vi "McPherson Set Scanning.vi"(0 "VISA Resource Name":refnum<visa-resource-name>, 1 "Stop@End?":bool, 2 "BeginSteps":i32 min=-8388607 max=8388607, 3 "EndSteps":i32 min=-8388607 max=8388607, 4 "Speed":i16, 5 "error In":errorcluster, 7 "Old Scan":bool, 8 "Scan":bool, 10 "Previous ScanStatus":T1, 13 "Pause":bool) -> (12 "dup VISA Resource Name":refnum<visa-resource-name>, 14 "Continue?":bool, 16 "ScanStatus Out":T1, 18 "Speed out":i32 min=-100000 max=100000, 19 "error out":errorcluster)   [LabVIEW 2020]
uses:
  McPhersonStatus.ctl
  Globals and TypeDefs/gSpectrometer.vi
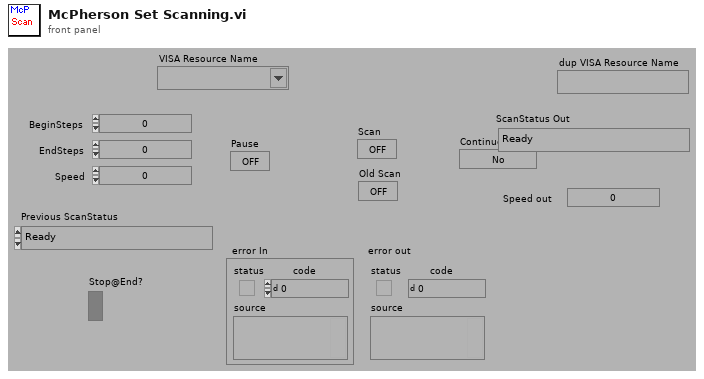
[diagram p1: front panel]
types:
  T1 = typedef "McPhersonStatus.ctl" = enum16{"Ready", "+Slew", "-Slew", "Slew Done", "Begin Scan", "+Slew to Start", "-Slew to Start", "Scanning", "Scan Done", "Scan Pause", "Slew Pause"}
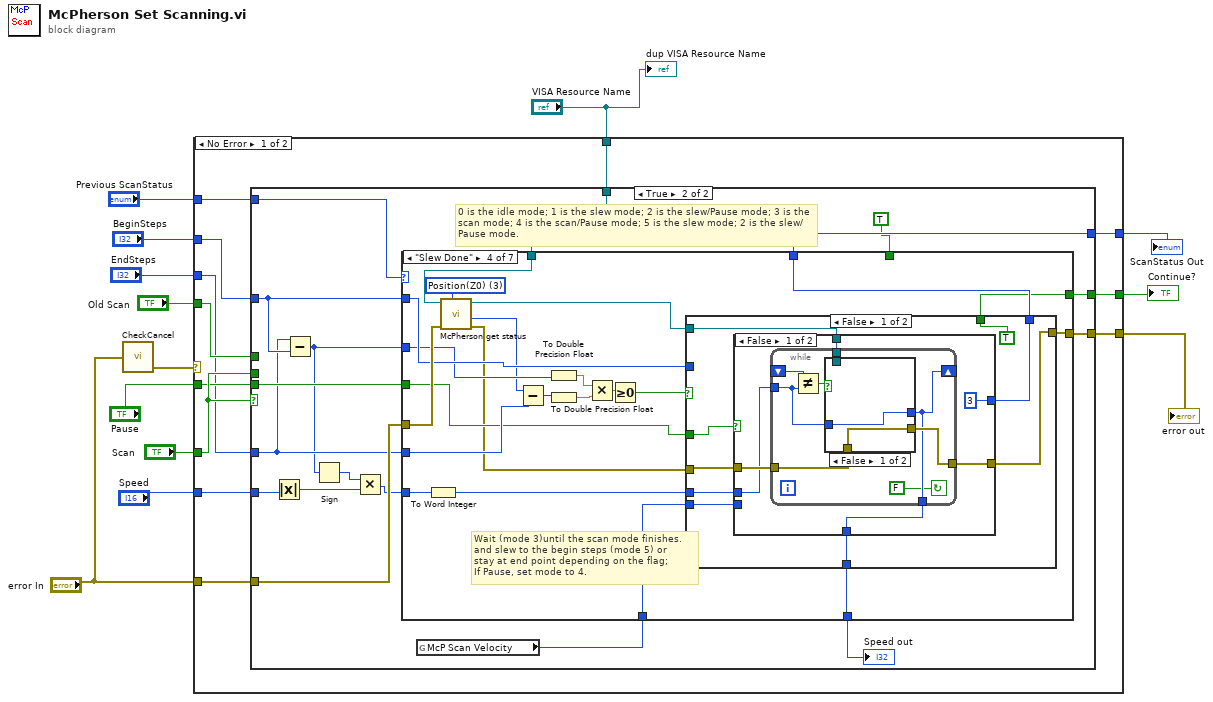
[diagram p0: block diagram]
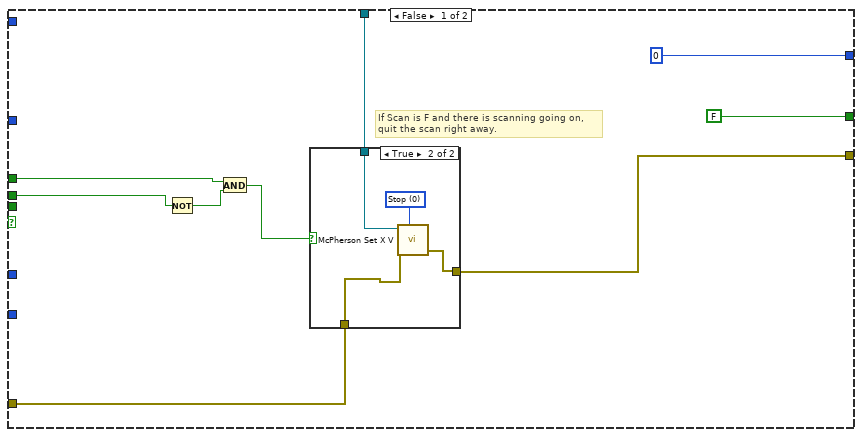
[diagram p2: hidden frame]
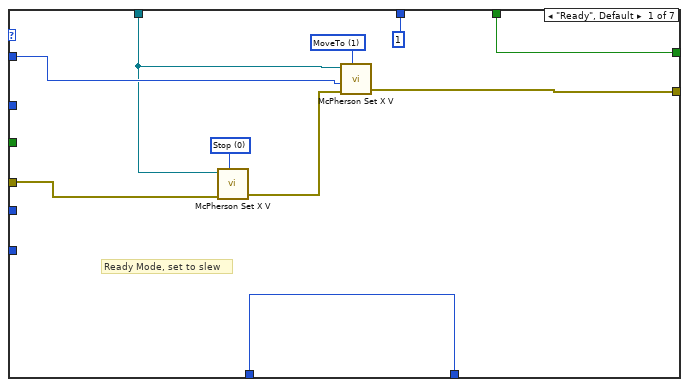
[diagram p4: hidden frame]
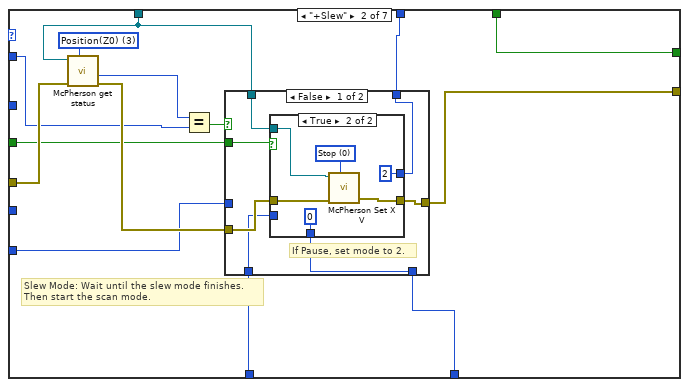
[diagram p5: hidden frame]
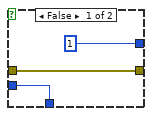
[diagram p6: hidden frame]
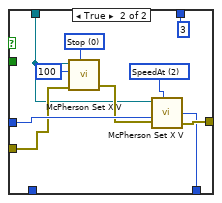
[diagram p7: hidden frame]
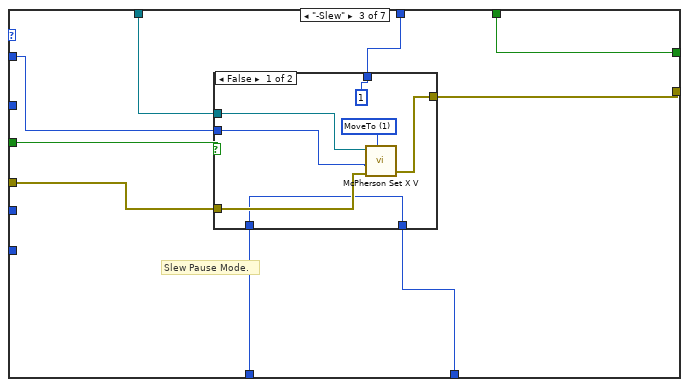
[diagram p8: hidden frame]
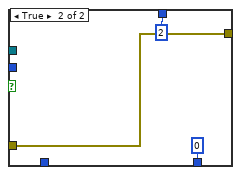
[diagram p9: hidden frame]
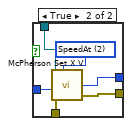
[diagram p10: hidden frame]
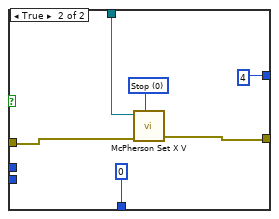
[diagram p11: hidden frame]
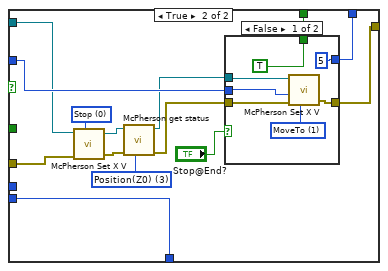
[diagram p12: hidden frame]
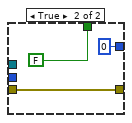
[diagram p13: hidden frame]
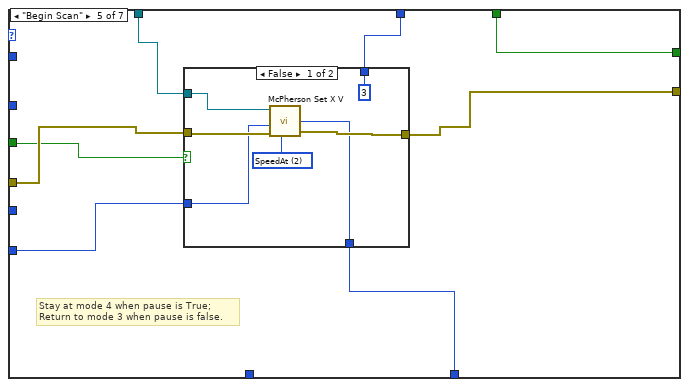
[diagram p14: hidden frame]
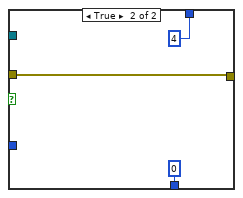
[diagram p15: hidden frame]
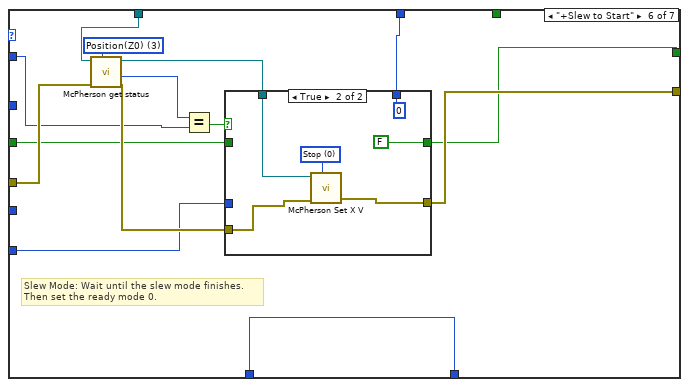
[diagram p16: hidden frame]
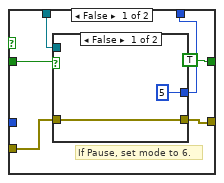
[diagram p17: hidden frame]
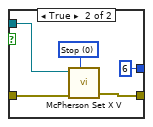
[diagram p18: hidden frame]
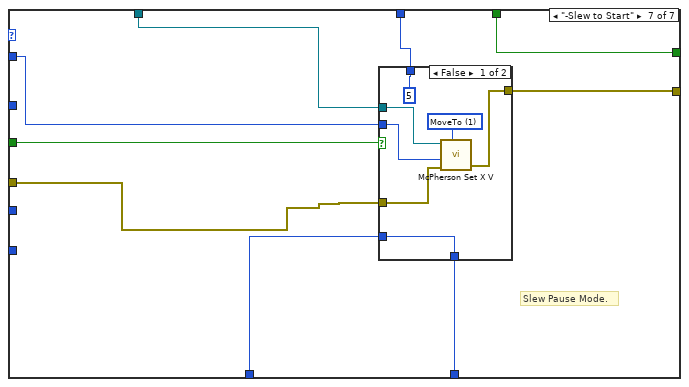
[diagram p19: hidden frame]
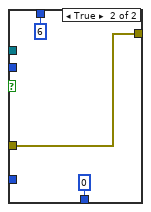
[diagram p20: hidden frame]
diagram:
  n1 = call "CheckCancel.vi"("error in (no error)"="error In") -> ("error out"=w2:errorcluster)  [unwired: 1 in, 1 out]
  n2 = case shown="No Error" w2 {
    tunnel: "VISA Resource Name" -> [w25 _]
    tunnel: "Scan" -> [w24 _]
    tunnel: "Old Scan" -> [w23 w279]
    tunnel: [w22 w279] -> w11
    tunnel: "Pause" -> [w18 _]
    tunnel: "Previous ScanStatus" -> [w21 w281]
    tunnel: [w20 w281] -> w4
    tunnel: "Speed" -> [w19 _]
    tunnel: "BeginSteps" -> [w17 _]
    tunnel: "EndSteps" -> [w16 _]
    tunnel: "error In" -> [w15 w280]
    tunnel: [w14 w280] -> w5
    frame No Error {
      n3 = case shown="True" w24 {
        tunnel: w17 -> [_ w46]
        tunnel: w16 -> [_ w45]
        tunnel: w25 -> [w33 w56]
        tunnel: w19 -> [_ w44]
        tunnel: w15 -> [w32 w55]
        tunnel: [w31 w54] -> w14
        tunnel: [FALSE w53] -> w22
        tunnel: w24 -> [w30 _]
        tunnel: w23 -> [w28 _]
        tunnel: w21 -> [_ w51]
        tunnel: [u8 0 ("ScanStatus") w50] -> w20
        tunnel: w18 -> [_ w49]
        frame False {
          # "If Scan is F and there is scanning going on,\nquit the scan right away."
          n4 = Not(x=w30) -> (.not. x?=w29:bool)
          n5 = And(x=w28, y=w29) -> (x .and. y?=w27:bool)
          n6 = case shown="True" w27 {
            tunnel: w33 -> [_ w39]
            tunnel: w32 -> [w35 w38]
            tunnel: [w35 w37] -> w31
            frame False {
            }
            frame True {
              w36 = u8 0 items=["Stop", "MoveTo", "SpeedAt"] ("Action")
              n7 = call "McPherson Set X V.vi"("VISA Resource Name"=w39, "error In"=w38, "Action"=w36) -> ("error out"=w37:errorcluster)  [unwired: 2 in, 2 out]
            }
          }
        }
        frame True {
          # "0 is the idle mode; 1 is the slew mode; 2 is the slew/Pause mode; 3 is the scan mode; 4 is the scan/Pause mode; 5 is the slew mode; 2 is the slew/Pause mode."
          n8 = Absolute Value(x=w44) -> (abs(x)=w48:i16)
          n9 = Subtract(x=w45, y=w46) -> (x-y=w42:i32)
          n10 = Sign(1:w42) -> (0:w47:i32)
          n11 = Multiply(x=w47, y=w48) -> (x*y=w43:i32)
          n12 = global read "gSpectrometer.vi" "McP Scan Velocity"() -> (w40:i32)
          n13 = case shown="\"Slew Done\"" w51 {
            tunnel: w56 -> [w58 w67 w114 w127 w216 w228 w267]
            tunnel: w46 -> [w62 w76 w115 w145 _ w236 w268]
            tunnel: w45 -> [_ _ _ w144 _ _ _]
            tunnel: w43 -> [_ w75 _ w131 w213 w235 _]
            tunnel: w55 -> [w60 w79 w110 w146 w215 w239 w263]
            tunnel: [w63 w80 w113 w143 w214 w240 w266] -> w54
            tunnel: [w64 w72 w109 w132 w210 w232 w262] -> w53
            tunnel: [w65 w70 w107 w134 w209 w231 w261] -> w52
            tunnel: [u8 1 ("ScanStatus") w73 w112 w139 w211 w233 w265] -> w50
            tunnel: w49 -> [_ w74 w111 w136 w212 w234 w264]
            tunnel: w42 -> [_ _ _ w138 _ _ _]
            tunnel: w40 -> [w65 w71 w108 w133 _ w231 w260]
            tunnel: TRUE ("Ramp") -> [w64 w72 w109 _ w210 _ w262]
            frame "Ready", Default {
              w57 = u8 0 items=["Stop", "MoveTo", "SpeedAt"] ("Action")
              w61 = u8 1 items=["Stop", "MoveTo", "SpeedAt"] ("Action")
              # "Ready Mode, set to slew"
              n14 = call "McPherson Set X V.vi"("VISA Resource Name"=w58, "error In"=w60, "Action"=w57) -> ("error out"=w59:errorcluster)  [unwired: 2 in, 2 out]
              n15 = call "McPherson Set X V.vi"("VISA Resource Name"=w58, "SetValue In"=w62, "error In"=w59, "Action"=w61) -> ("error out"=w63:errorcluster)  [unwired: 1 in, 2 out]
            }
            frame "+Slew" {
              w68 = u16 3 items=["Grab Globals", "Full (X, ^, Z0)", "Moving(^ and Z0)", "Position(Z0)"] ("Status")
              # "Slew Mode: Wait until the slew mode finishes.\nThen start the scan mode."
              n16 = call "McPherson get status.vi"("Status"=w68, "error in (no error)"=w79, "VISA Resource Name"=w67) -> ("error out"=w78:errorcluster, "CurrentPosition"=w69:i32)  [unwired: 2 in, 2 out]
              n17 = Equal?(x=w69, y=w76) -> (x = y?=w77:bool)
              n18 = case shown="False" w77 {
                tunnel: w67 -> [w83 w99]
                tunnel: w75 -> [_ w106]
                tunnel: w78 -> [w84 w101]
                tunnel: [w85 w105] -> w80
                tunnel: [w81 w104] -> w70
                tunnel: [w86 u8 3 ("ScanStatus")] -> w73
                tunnel: w74 -> [w87 _]
                tunnel: w71 -> [w82 _]
                frame False {
                  # "If Pause, set mode to 2."
                  n19 = case shown="True" w87 {
                    tunnel: [u8 1 ("ScanStatus") u8 2 ("ScanStatus")] -> w86
                    tunnel: [w89 w96] -> w85
                    tunnel: w84 -> [w89 w95]
                    tunnel: w83 -> [_ w93]
                    tunnel: w82 -> [w88 _]
                    tunnel: [w88 0 ("McP Scan Velocity")] -> w81
                    frame False {
                    }
                    frame True {
                      w92 = u8 0 items=["Stop", "MoveTo", "SpeedAt"] ("Action")
                      n20 = call "McPherson Set X V.vi"("VISA Resource Name"=w93, "error In"=w95, "Action"=w92) -> ("error out"=w96:errorcluster)  [unwired: 2 in, 2 out]
                    }
                  }
                }
                frame True {
                  w98 = u8 0 items=["Stop", "MoveTo", "SpeedAt"] ("Action")
                  w102 = u8 2 items=["Stop", "MoveTo", "SpeedAt"] ("Action")
                  n21 = call "McPherson Set X V.vi"("VISA Resource Name"=w99, "milliseconds to wait"=u32 100, "error In"=w101, "Action"=w98) -> ("error out"=w100:errorcluster)  [unwired: 1 in, 2 out]
                  n22 = call "McPherson Set X V.vi"("VISA Resource Name"=w99, "SetValue In"=w106, "error In"=w100, "Action"=w102) -> ("SetValue Out"=w104:i32, "error out"=w105:errorcluster)  [unwired: 1 in, 1 out]
                }
              }
            }
            frame "-Slew" {
              # "Slew Pause Mode."
              n23 = case shown="False" w111 {
                tunnel: w115 -> [w118 _]
                tunnel: w114 -> [w119 _]
                tunnel: [w122 w125] -> w113
                tunnel: [u8 1 ("ScanStatus") u8 2 ("ScanStatus")] -> w112
                tunnel: w110 -> [w120 w125]
                tunnel: [w116 0 ("McP Scan Velocity")] -> w107
                tunnel: w108 -> [w116 _]
                frame False {
                  w117 = u8 1 items=["Stop", "MoveTo", "SpeedAt"] ("Action")
                  n24 = call "McPherson Set X V.vi"("VISA Resource Name"=w119, "SetValue In"=w118, "error In"=w120, "Action"=w117) -> ("error out"=w122:errorcluster)  [unwired: 1 in, 2 out]
                }
                frame True {
                }
              }
            }
            frame "Slew Done" {
              w129 = u16 3 items=["Grab Globals", "Full (X, ^, Z0)", "Moving(^ and Z0)", "Position(Z0)"] ("Status")
              # "Wait (mode 3)until the scan mode finishes.\nand slew to the begin steps (mode 5) or\nstay at end point depending on the flag;\nIf Pause, set mode to 4."
              n25 = To Word Integer(number=w131) -> (16bit integer=w130:i16)
              n26 = call "McPherson get status.vi"("Status"=w129, "error in (no error)"=w146, "VISA Resource Name"=w127) -> ("error out"=w135:errorcluster, "CurrentPosition"=w128:i32, "dup VISA Resource Name"=w126:refnum<visa-resource-name>)  [unwired: 2 in, 1 out]
              n27 = Subtract(x=w128, y=w144) -> (x-y=w142:i32)
              n28 = To Double Precision Float(number=w138) -> (double precision float=w140:dbl)
              n29 = To Double Precision Float(number=w142) -> (double precision float=w141:dbl)
              n30 = Multiply(x=w140, y=w141) -> (x*y=w147:dbl)
              n31 = Greater Or Equal To 0?(x=w147) -> (x >= 0?=w137:bool)
              n32 = case shown="False" w137 {
                tunnel: w145 -> [_ w198]
                tunnel: w126 -> [w153 w188]
                tunnel: w135 -> [w156 w191]
                tunnel: [w155 w197] -> w143
                tunnel: [w151 w195] -> w139
                tunnel: w136 -> [w152 _]
                tunnel: w130 -> [w154 _]
                tunnel: [w150 w194] -> w134
                tunnel: w133 -> [w149 w194]
                tunnel: [TRUE ("Ramp") w193] -> w132
                frame False {
                  n33 = case shown="False" w152 {
                    tunnel: w156 -> [w162 w183]
                    tunnel: [w161 w182] -> w155
                    tunnel: w154 -> [w160 _]
                    tunnel: w153 -> [w159 w181]
                    tunnel: [u8 3 ("ScanStatus") u8 4 ("t")] -> w151
                    tunnel: [w157 0 ("McP Scan Velocity")] -> w150
                    tunnel: w149 -> [_ _]
                    frame False {
                      n34 = while {
                        shift-left: _ -> [w166]
                        shift-right: [w167] -> _
                        tunnel: w160 -> [w164]
                        tunnel: [w167] -> w157
                        tunnel: [w168] -> w161
                        tunnel: w159 -> [w169]
                        tunnel: w162 -> [w170]
                        stop <- FALSE continue-if-true
                        n35 = Not Equal?(x=w166, y=w164) -> (x != y?=w165:bool)
                        n36 = case shown="False" w165 {
                          tunnel: w170 -> [w172 w178]
                          tunnel: w169 -> [_ w177]
                          tunnel: [w172 w176] -> w168
                          tunnel: [w171 w175] -> w167
                          tunnel: w164 -> [w171 w174]
                          frame False {
                          }
                          frame True {
                            w173 = u8 2 items=["Stop", "MoveTo", "SpeedAt"] ("Action")
                            n37 = call "McPherson Set X V.vi"("VISA Resource Name"=w177, "SetValue In"=w174, "error In"=w178, "Action"=w173) -> ("SetValue Out"=w175:i32, "error out"=w176:errorcluster)  [unwired: 1 in, 1 out]
                          }
                        }
                      }
                    }
                    frame True {
                      w180 = u8 0 items=["Stop", "MoveTo", "SpeedAt"] ("Action")
                      n38 = call "McPherson Set X V.vi"("VISA Resource Name"=w181, "error In"=w183, "Action"=w180) -> ("error out"=w182:errorcluster)  [unwired: 2 in, 2 out]
                    }
                  }
                }
                frame True {
                  w187 = u16 3 items=["Grab Globals", "Full (X, ^, Z0)", "Moving(^ and Z0)", "Position(Z0)"] ("Status")
                  w192 = u8 0 items=["Stop", "MoveTo", "SpeedAt"] ("Action")
                  n39 = call "McPherson Set X V.vi"("VISA Resource Name"=w188, "error In"=w191, "Action"=w192) -> ("dup VISA Resource Name"=w186:refnum<visa-resource-name>, "error out"=w189:errorcluster)  [unwired: 2 in, 1 out]
                  n40 = call "McPherson get status.vi"("Status"=w187, "error in (no error)"=w189, "VISA Resource Name"=w186) -> ("error out"=w190:errorcluster, "dup VISA Resource Name"=w185:refnum<visa-resource-name>)  [unwired: 2 in, 2 out]
                  n41 = case shown="False" "Stop@End?" {
                    tunnel: w198 -> [w203 _]
                    tunnel: w185 -> [w200 _]
                    tunnel: w190 -> [w199 w207]
                    tunnel: [w205 w207] -> w197
                    tunnel: [u8 5 ("ScanStatus") u8 0 ("ScanStatus")] -> w195
                    tunnel: [TRUE ("Ramp") FALSE ("Ramp")] -> w193
                    frame False {
                      w202 = u8 1 items=["Stop", "MoveTo", "SpeedAt"] ("Action")
                      n42 = call "McPherson Set X V.vi"("VISA Resource Name"=w200, "SetValue In"=w203, "error In"=w199, "Action"=w202) -> ("error out"=w205:errorcluster)  [unwired: 1 in, 2 out]
                    }
                    frame True {
                    }
                  }
                }
              }
            }
            frame "Begin Scan" {
              # "Stay at mode 4 when pause is True;\nReturn to mode 3 when pause is false."
              n43 = case shown="False" w212 {
                tunnel: w216 -> [w221 _]
                tunnel: w215 -> [w222 w226]
                tunnel: [w219 w226] -> w214
                tunnel: w213 -> [w220 _]
                tunnel: [u8 3 ("ScanStatus") u8 4 ("ScanStatus")] -> w211
                tunnel: [w218 0 ("ScanSpeed Out")] -> w209
                frame False {
                  w217 = u8 2 items=["Stop", "MoveTo", "SpeedAt"] ("Action")
                  n44 = call "McPherson Set X V.vi"("VISA Resource Name"=w221, "SetValue In"=w220, "error In"=w222, "Action"=w217) -> ("SetValue Out"=w218:i32, "error out"=w219:errorcluster)  [unwired: 1 in, 1 out]
                }
                frame True {
                }
              }
            }
            frame "+Slew to Start" {
              w230 = u16 3 items=["Grab Globals", "Full (X, ^, Z0)", "Moving(^ and Z0)", "Position(Z0)"] ("Status")
              # "Slew Mode: Wait until the slew mode finishes.\nThen set the ready mode 0."
              n45 = call "McPherson get status.vi"("Status"=w230, "error in (no error)"=w239, "VISA Resource Name"=w228) -> ("error out"=w238:errorcluster, "CurrentPosition"=w229:i32, "dup VISA Resource Name"=w227:refnum<visa-resource-name>)  [unwired: 2 in, 1 out]
              n46 = Equal?(x=w229, y=w236) -> (x = y?=w237:bool)
              n47 = case shown="True" w237 {
                tunnel: w227 -> [w242 w256]
                tunnel: w235 -> [_ _]
                tunnel: w238 -> [w243 w255]
                tunnel: [w244 w254] -> w240
                tunnel: [w245 u8 0 ("ScanStatus")] -> w233
                tunnel: w234 -> [w246 _]
                tunnel: [TRUE ("Ramp") FALSE ("Ramp")] -> w232
                frame False {
                  # "If Pause, set mode to 6."
                  n48 = case shown="False" w246 {
                    tunnel: [u8 5 ("ScanStatus") u8 6 ("ScanStatus")] -> w245
                    tunnel: [w247 w253] -> w244
                    tunnel: w243 -> [w247 w252]
                    tunnel: w242 -> [_ w250]
                    frame False {
                    }
                    frame True {
                      w249 = u8 0 items=["Stop", "MoveTo", "SpeedAt"] ("Action")
                      n49 = call "McPherson Set X V.vi"("VISA Resource Name"=w250, "error In"=w252, "Action"=w249) -> ("error out"=w253:errorcluster)  [unwired: 2 in, 2 out]
                    }
                  }
                }
                frame True {
                  w257 = u8 0 items=["Stop", "MoveTo", "SpeedAt"] ("Action")
                  n50 = call "McPherson Set X V.vi"("VISA Resource Name"=w256, "error In"=w255, "Action"=w257) -> ("error out"=w254:errorcluster)  [unwired: 2 in, 2 out]
                }
              }
            }
            frame "-Slew to Start" {
              # "Slew Pause Mode."
              n51 = case shown="False" w264 {
                tunnel: w268 -> [w271 _]
                tunnel: w267 -> [w272 _]
                tunnel: [w275 w278] -> w266
                tunnel: [u8 5 ("ScanStatus") u8 6 ("ScanStatus")] -> w265
                tunnel: w263 -> [w273 w278]
                tunnel: [w269 0 ("McP Scan Velocity")] -> w261
                tunnel: w260 -> [w269 _]
                frame False {
                  w270 = u8 1 items=["Stop", "MoveTo", "SpeedAt"] ("Action")
                  n52 = call "McPherson Set X V.vi"("VISA Resource Name"=w272, "SetValue In"=w271, "error In"=w273, "Action"=w270) -> ("error out"=w275:errorcluster)  [unwired: 1 in, 2 out]
                }
                frame True {
                }
              }
            }
          }
          "Speed out" <- w52
        }
      }
    }
    frame Error {
    }
  }
  "ScanStatus Out" <- w4
  "Continue?" <- w11
  "error out" <- w5
  "dup VISA Resource Name" <- "VISA Resource Name"
